vi "Test Compare Enums Generates Message.vi"(8 "error in (no error)":errorcluster, 11 "Compare Assertion Test In":refnum<class "Compare Assertion Test.lvclass">) -> (0 "error out":errorcluster, 3 "Compare Assertion Test Out":refnum<class "Compare Assertion Test.lvclass">)   [LabVIEW 2020, in "LUnit Tests.lvlib" / "Compare Assertion Test.lvclass"]
uses:
  Compare Assertion Test.lvclass
  C:/Program Files (x86)/National Instruments/LabVIEW 2020/vi.lib/Astemes/LUnit/Test Case.lvclass
  Test Dummys/Test Case Test Double/Test Case Test Double.lvclass
  <vilib>/Astemes/LUnit/Test Case.lvclass/Test Case.ctl
  85eca79f-c10f-4dc8-9635-a30d13beb79f.vi
  <vilib>/Astemes/LUnit/Palette/Pass.vi
  <vilib>/Astemes/LUnit/Palette/Fail.vi
  <vilib>/Astemes/LUnit/Compare Variants.vi
  <vilib>/Astemes/LUnit/Describe Comparison.vi
  <vilib>/Astemes/LUnit/Set Assertion Type.vi
  <vilib>/Astemes/LUnit/Add test result.vi
  <vilib>/Astemes/LUnit/Variant to string.vi
  <vilib>/Astemes/LUnit/LUnit Record Assertion Result.vi
  <vilib>/Astemes/LUnit/LUnit Aggregate Assertion Results.vi
  <vilib>/Astemes/LUnit/Method Result/LUnit Merge Status.vi
  <vilib>/Astemes/LUnit/LUnit Concatenate result strings.vi
  <vilib>/Utility/Data Type/Get Type Information.vi
  <vilib>/Utility/LVClass/Get LV Class Name.vi
  Compare Assertion Test.lvclass/Compare Assertion Test.ctl
panel:
  out "Message":string
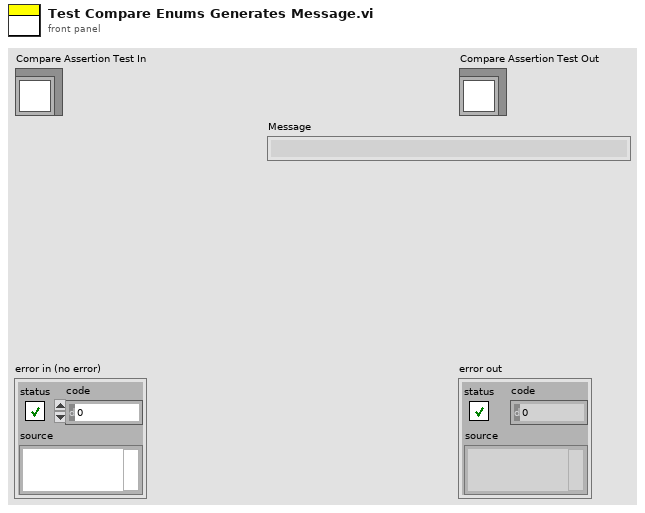
[diagram p1: front panel]
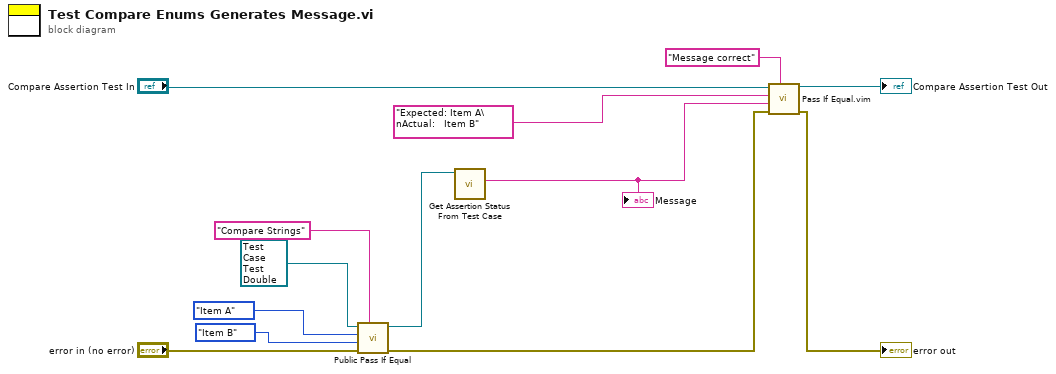
[diagram p0: block diagram]
diagram:
  n1 = call "Public Pass If Equal.vi"("Description"="Compare Strings", "error in (no error)"="error in (no error)", "Actual"=enum16{"Item A", "Item B"}."Item B", "Expected"=enum16{"Item A", "Item B"}."Item A", "Test Case Test Double in"=refnum<class "Test Case Test Double.lvclass"> refnum ("Test Case Test Double.lvclass")) -> ("error out"=w11:errorcluster, "Test Case Test Double out"=w10:refnum<class "Test Case Test Double.lvclass">)  [unwired: 5 in]
  n2 = call "Get Assertion Status From Test Case.vi"("Test Case Test Double in"=w10) -> ("Message"=w2:string)  [unwired: 9 in, 1 out]
  "Message" <- w2
  n3 = call "Pass If Equal.vim"("Description"="Message correct", "error in (no error)"=w11, "Actual"=w2, "Expected"="Expected: Item A\nActual:   Item B", "LUnit Test Case In"="Compare Assertion Test In") -> ("error out"=→"error out":errorcluster, "LUnit Test Case Out"=→"Compare Assertion Test Out":refnum<class "Compare Assertion Test.lvclass">)  [unwired: 5 in]
